vi "Get CDO Configuration.vi"(8 "error in":errorcluster, 10 "channels":refnum<class "Channel.lvclass">[](array[class]), 11 "counter driven output mode in":refnum<class "Counter Driven Output Mode.lvclass">) -> (0 "error out":errorcluster, 2 "CDO":T1, 3 "counter driven output mode out":refnum<class "Counter Driven Output Mode.lvclass">)   [LabVIEW 2017, in "Scan Engine Scripting.lvlib" / "Counter Driven Output Mode.lvclass"]
uses:
  Counter Driven Output Mode.lvclass
  Channel Classes/Channel/Channel.lvclass
  Channel Classes/Counter Driven Output Channel/Counter Driven State.ctl
  Channel Classes/Counter Driven Output Channel/Counter Driven Output Channel.lvclass
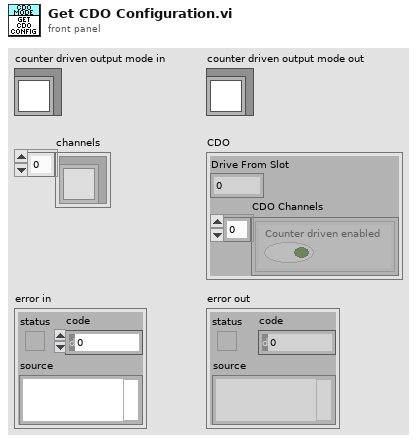
[diagram p1: front panel]
types:
  T1 = cluster{"Drive From Slot":u32, "CDO Channels":cluster{"Counter driven enabled":bool}[]}
  T2 = typedef "Scan Engine Scripting.lvlib/Counter Driven Output Mode.lvclass/Drive from Slot.ctl" = enum16{"Slot 1", "Slot 2", "Slot 3", "Slot 4", "Slot 5", "Slot 6", "Slot 7", "Slot 8"}
  T3 = typedef "Scan Engine Scripting.lvlib/counter driven output channel settings.ctl" = cluster{"name":string, "default value":bool, "counter driven state":T4}
  T4 = typedef "Scan Engine Scripting.lvlib/Counter Driven Output Channel.lvclass/Counter Driven State.ctl" = enum16{"Disabled", "Enabled"}
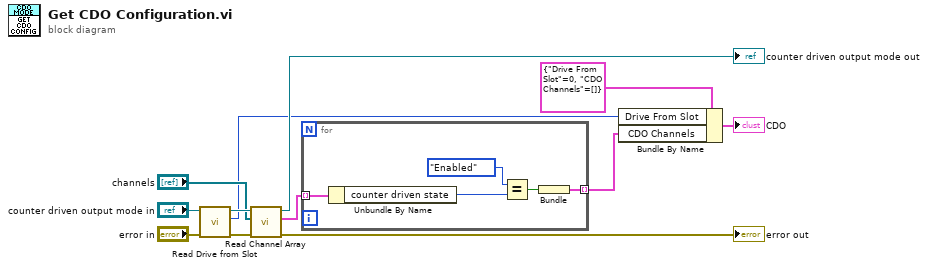
[diagram p0: block diagram]
diagram:
  n1 = call-dynamic "Read Drive from Slot.vi"("error in"="error in", "counter driven output mode in"="counter driven output mode in") -> ("error out"=w6:errorcluster, "drive from slot"=w5:T2, "counter driven output mode out"=w12:refnum<class "Counter Driven Output Mode.lvclass">)  [unwired: 7 in]
  n2 = call "Read Channel Array.vi"("error in"=w6, "channels"="channels", "counter driven output mode in"=w12) -> ("error out"=→"error out":errorcluster, "channel settings"=w3:T3[], "counter driven output mode out"=→"counter driven output mode out":refnum<class "Counter Driven Output Mode.lvclass">)  [unwired: 6 in]
  n3 = for {
    tunnel: w3 -> [w17] mode=indexing
    tunnel: [w13] -> w1 mode=indexing
    n4 = Unbundle By Name(w17) -> ("counter driven state"=w15:T4)
    n5 = Equal?(x=Counter_Driven_State."Enabled", y=w15) -> (x = y?=w14:bool)
    n6 = Bundle(w14) -> (w13:cluster{bool})  [unwired: 1 in]
  }
  n7 = Bundle By Name(cluster=T1 {"Drive From Slot"=0, "CDO Channels"=[]} ("CDO"), "Drive From Slot"=w5, "CDO Channels"=w1) -> (→"CDO":T1)
